vi "Read Current Excitation Value.vi"(8 "error in (no error)":errorcluster, 11 "BNT_DMQmx-MCSV-RTD in":refnum<class "BNT_DAQmx-MCSV-RTD.lvclass">) -> (0 "error out":errorcluster, 2 "Current Excitation Value":dbl=0.0025 format="%0.5f", 3 "BNT_DMQmx-MCSV-RTD out":refnum<class "BNT_DAQmx-MCSV-RTD.lvclass">)   [LabVIEW 2017, in "BNT_DAQmx.lvlib" / "BNT_DAQmx-MCSV-RTD.lvclass"]
doc: "Read Current Excitation Value."
uses:
  BNT_DAQmx-MCSV-RTD.lvclass
  BNT_DAQmx-MCSV-RTD.lvclass/BNT_DAQmx-MCSV-RTD.ctl
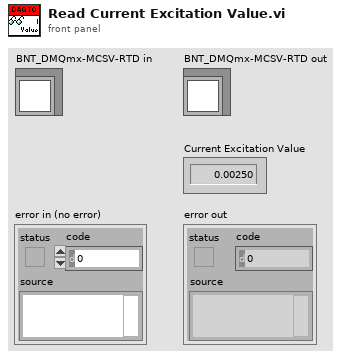
[diagram p1: front panel]
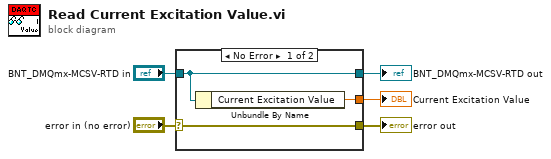
[diagram p0: block diagram]
diagram:
  n1 = case shown="No Error" "error in (no error)" {
    selector: "error in (no error)" -> [w8 w9]
    tunnel: [w8 w9] -> w4
    tunnel: [w7 w10] -> w2
    tunnel: "BNT_DMQmx-MCSV-RTD in" -> [w7 w10]
    tunnel: [w6 _] -> w1
    frame No Error {
      n2 = Unbundle By Name(w7) -> ("Current Excitation Value"=w6:dbl)
    }
    frame Error {
    }
  }
  "error out" <- w4
  "BNT_DMQmx-MCSV-RTD out" <- w2
  "Current Excitation Value" <- w1
